vi "Screen Capture.vi"() -> ()   [LabVIEW 2013]
doc: "This VI captures the region of the screen and displays it on the front panel continuously.\nCan be used to develop remote desktop applications."
uses:
  <vilib>/Utility/miscctls.llb/LVBoundsTypeDef.ctl
  System.Drawing
  <vilib>/Utility/inputDevices.llb/closeMouse.vi
  <vilib>/Utility/inputDevices.llb/mouseAcquire.vi
  <vilib>/wsapi/NI_WebServices.lvlib
panel:
  in  "Height (px)":i32=100
  in  "Width (px)":i32=100
  out "Screen Capture":picture
  in  "stop":bool
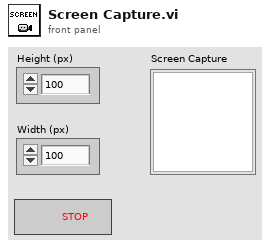
[diagram p1: front panel]
types:
  T1 = typedef "LVBoundsTypeDef.ctl" = cluster{"Width":u32, "Height":u32}
  T2 = cluster{"Horizontal":i32, "Vertical":i32, "Scrolling":i32}
  T3 = typedef "imagedata.ctl" = cluster{"image type":i32, "image depth":i32, "image":u8[], "mask":u8[], "colors":u32[], "Rectangle":cluster{"left":i16, "top":i16, "right":i16, "bottom":i16}}
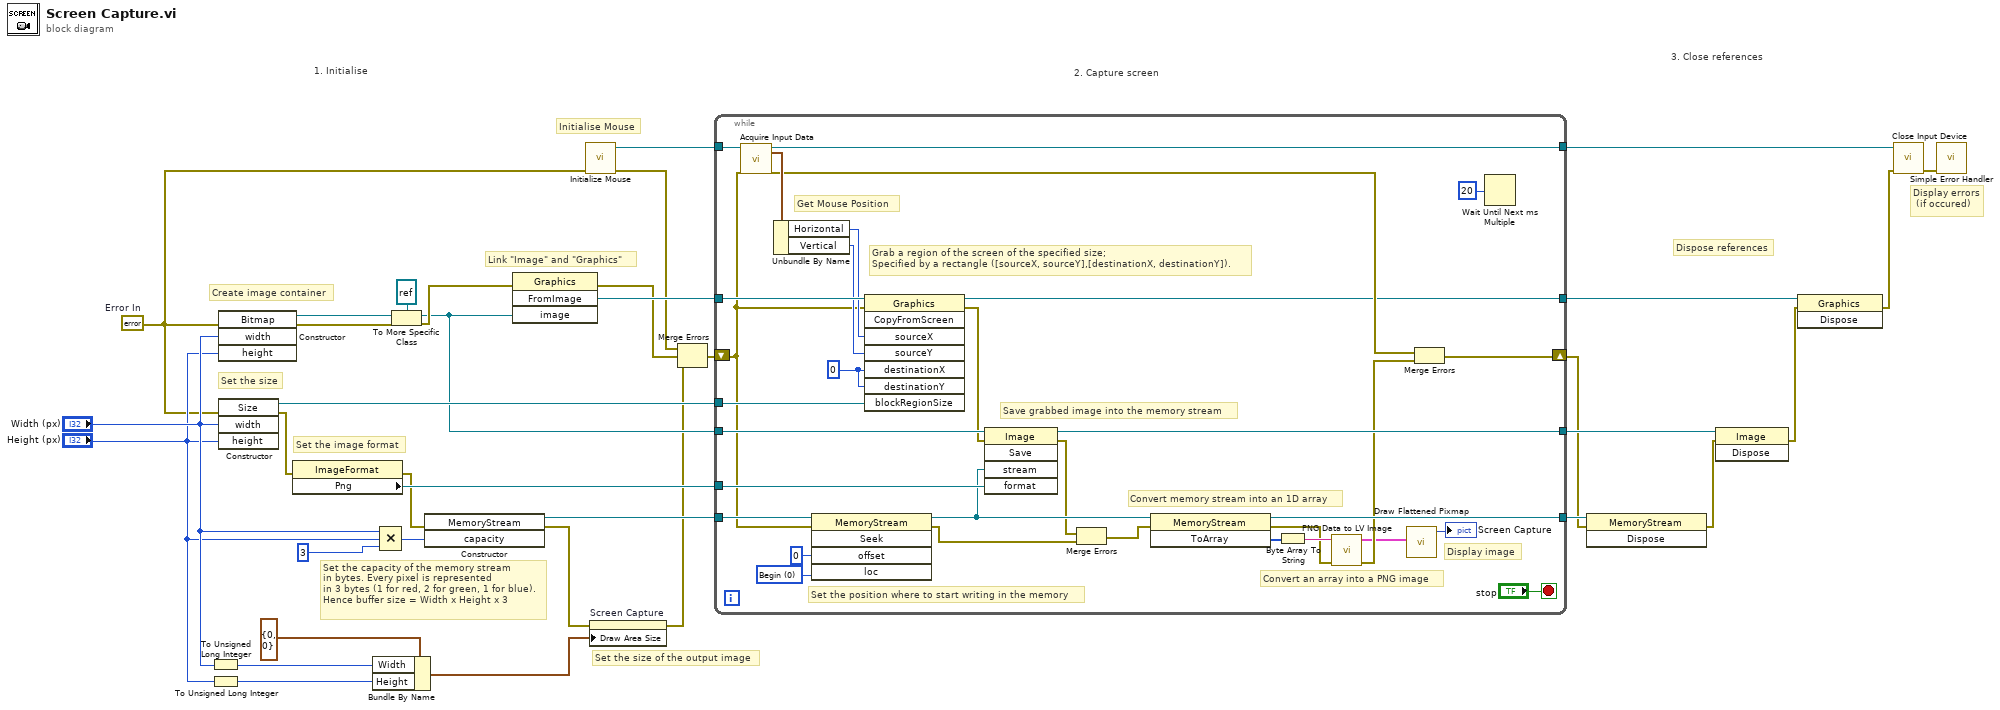
[diagram p0: block diagram]
diagram:
  w1 = errorcluster {"status"=FALSE, "code"=0, "source"=""}  # Error In
  # "Link \"Image\" and \"Graphics\""
  # "Set the size"
  # "Create image container"
  # "3. Close references"
  # "2. Capture screen"
  # "1. Initialise"
  # "Display errors\n (if occured)"
  # "Dispose references"
  # "Set the image format"
  # "Set the size of the output image"
  # "Set the capacity of the memory stream\nin bytes. Every pixel is represented\nin 3 bytes (1 for red, 2 for green, 1 for blue).\nHence buffer size = Width x Height x 3"
  # "Initialise Mouse"
  n1 = To Unsigned Long Integer(number="Width (px)") -> (unsigned 32bit integer=w9:u32)
  n2 = To Unsigned Long Integer(number="Height (px)") -> (unsigned 32bit integer=w7:u32)
  n3 = constructor class="Bitmap"(error in=w1, "width"="Width (px)", "height"="Height (px)") -> (reference out=w29:refnum<k24>, error out=w32:errorcluster)  [unwired: 2 in, 3 out]
  n4 = constructor class="Size"(error in=w1, "width"="Width (px)", "height"="Height (px)") -> (reference out=w27:refnum<k24>, error out=w18:errorcluster)  [unwired: 2 in, 3 out]
  n5 = property class="ImageFormat"(error in=w18) -> (error out=w17:errorcluster, "Png"=w26:refnum<k24>)  [unwired: 1 in, 1 out]
  n6 = Bundle By Name(cluster=T1 {"Width"=0, "Height"=0} ("Draw Area Size"), "Width"=w9, "Height"=w7) -> (w13:T1)
  n7 = Compound Arithmetic op=MULTIPLY("Width (px)", "Height (px)", 3 ("value")) -> (w21:i32)
  n8 = To More Specific Class(target class=refnum<k24> refnum, reference=w29, error in=w32) -> (specific class reference=w20:refnum<k24>, error out=w33:errorcluster)
  n9 = constructor class="MemoryStream"(error in=w17, "capacity"=w21) -> (reference out=w23:refnum<k24>, error out=w12:errorcluster)  [unwired: 2 in, 2 out]
  n10 = invoke class="Graphics" method="FromImage"(error in=w33, "image"=w20) -> (error out=w16:errorcluster, "FromImage"=w30:refnum<k24>)  [unwired: 2 in, 2 out]
  n11 = call <vilib>:"Initialize Mouse.vi"("error in (no error)"=w1) -> ("error out"=w14:errorcluster, "device ID"=w35:refnum<k1>)  [unwired: 9 in]
  n12 = property on="Screen Capture" class="Pict"(error in=w12, "Draw Area Size"=w13) -> (error out=w11:errorcluster)  [unwired: 1 in, 1 out]
  n13 = Merge Errors(w14, w16, w11) -> (w15:errorcluster)
  n14 = while {
    tunnel: w35 -> [w67]
    tunnel: [w65] -> w34
    tunnel: w30 -> [w64]
    tunnel: [w61] -> w28
    tunnel: w27 -> [w60]
    tunnel: w26 -> [w59]
    tunnel: [w58] -> w25
    tunnel: w23 -> [w57]
    tunnel: w20 -> [w50]
    shift-right: [w39] -> w6
    shift-left: w15 -> [w42]
    tunnel: [w38] -> w5
    stop <- "stop" stop-if-true
    w51 = 0 ("destinationX")
    w55 = 0 items=["Begin", "Current", "End"] ("loc")
    # "Display image"
    # "Convert an array into a PNG image"
    # "Set the position where to start writing in the memory"
    # "Convert memory stream into an 1D array"
    # "Save grabbed image into the memory stream"
    # "Grab a region of the screen of the specified size;\nSpecified by a rectangle ([sourceX, sourceY],[destinationX, destinationY])."
    # "Get Mouse Position"
    n15 = call-poly <vilib>:"Acquire Input Data.vi"("device ID"=w67, "error in (no error)"=w42) -> ("device ID"=w65:refnum<k1>, "axis info"=w66:T2, "error out"=w41:errorcluster)  [unwired: 14 in, 1 out]
    n16 = Unbundle By Name(w66) -> ("Horizontal"=w45:i32, "Vertical"=w44:i32)
    n17 = invoke class="MemoryStream" method="Seek"(reference=w57, error in=w42, "offset"=i64 0, "loc"=w55) -> (reference out=w52:refnum<k24>, error out=w47:errorcluster)  [unwired: 1 in, 3 out]
    n18 = invoke class="Graphics" method="CopyFromScreen"(reference=w64, error in=w42, "sourceX"=w45, "sourceY"=w44, "destinationX"=w51, "destinationY"=w51, "blockRegionSize"=w60) -> (reference out=w38:refnum<k24>, error out=w43:errorcluster)  [unwired: 1 in, 6 out]
    n19 = invoke class="Image" method="Save"(reference=w50, error in=w43, "stream"=w52, "format"=w59) -> (reference out=w58:refnum<k24>, error out=w48:errorcluster)  [unwired: 1 in, 3 out]
    n20 = Merge Errors(w48, w47) -> (w46:errorcluster)
    n21 = invoke class="MemoryStream" method="ToArray"(reference=w52, error in=w46) -> (reference out=w61:refnum<k24>, error out=w49:errorcluster, "ToArray"=w63:u8[])  [unwired: 1 in]
    n22 = Byte Array To String(unsigned byte array=w63) -> (string=w62:string)
    n23 = call <vilib>:"PNG Data to LV Image.vi"("error in (no error)"=w49, "png data"=w62) -> ("error out"=w40:errorcluster, "image data"=w37:T3)  [unwired: 8 in]
    n24 = call <vilib>:"Draw Flattened Pixmap.vi"("image data"=w37) -> ("new picture"=→"Screen Capture":picture)  [unwired: 8 in]
    n25 = Merge Errors(w41, w40) -> (w39:errorcluster)
    n26 = Wait Until Next ms Multiple(millisecond multiple=u32 20) -> ()  [unwired: 1 out]
  }
  n27 = invoke class="MemoryStream" method="Dispose"(reference=w28, error in=w6) -> (error out=w24:errorcluster)  [unwired: 1 in, 2 out]
  n28 = invoke class="Image" method="Dispose"(reference=w25, error in=w24) -> (error out=w4:errorcluster)  [unwired: 1 in, 2 out]
  n29 = invoke class="Graphics" method="Dispose"(reference=w5, error in=w4) -> (error out=w3:errorcluster)  [unwired: 1 in, 2 out]
  n30 = call-poly <vilib>:"Close Input Device.vi"("error in (no error)"=w3, "device ID"=w34) -> ("error out"=w2:errorcluster)  [unwired: 8 in]
  n31 = call <vilib>:"Simple Error Handler.vi"("error in (no error)"=w2) -> ()  [unwired: 4 in, 5 out]
